vi "Process.vi"(8 "error in":errorcluster, 11 "Inst UI.Framework-Template":refnum<class "Inst UI.Framework-Template.lvclass">) -> (0 "error out":errorcluster, 3 "Inst UI.Framework-Template out":refnum<class "Inst UI.Framework-Template.lvclass">)   [LabVIEW 2019, in "Inst UI.Framework-Template.lvclass"]
doc: "---------------------------------------------------------------\nJKI State Machine Objects™\nhttp://jki.net/state-machine-objects/\nCopyright (C) 2005-2015, JKI <info@jki.net>\nALL RIGHTS RESERVEDJKI State Machine Objects (SMO) 1.0.0.5\nJKI - JKI\nCopyright (c) 2016, JKI"
uses:
  Inst UI.Framework-Template.lvclass
  C:/Program Files (x86)/National Instruments/LabVIEW 2019/vi.lib/JKI/JKI SMO/SMO/SMO.lvclass
  C:/Program Files (x86)/National Instruments/LabVIEW 2019/user.lib/LevyLab/Instrument Framework/SMOs/Instrument UI/Instrument UI.lvclass
  C:/Program Files (x86)/National Instruments/LabVIEW 2019/vi.lib/JKI/JKI SMO/SMO.UI/SMO.UI.lvclass
  Inst.Framework-Template/Typedefs/Inst.Framework-Template.getAll--Cluster.ctl
  Inst.Framework-Template/Inst.Framework-Template.lvclass
  C:/Program Files (x86)/National Instruments/LabVIEW 2019/user.lib/LevyLab/Instrument Framework/SMOs/Instrument/Instrument.lvclass
  Inst UI.Framework-Template.UI--Cluster.ctl
  Inst.Framework-Template/Typedefs/Inst.Framework-Template.Configuration--Cluster.ctl
  <userlib>/LevyLab/Instrument Framework/SMOs/Configuration/Configuration.lvclass
  <userlib>/LevyLab/Instrument Framework/SMOs/RemoteControl/Typedefs/Message--Cluster.ctl
  <userlib>/LevyLab/Instrument Framework/SMOs/Instrument UI/Instrument UI.lvclass/Instrument UI.ctl
  Inst.Framework-Template/Inst.Framework-Template.lvclass/Inst.Framework-Template.ctl
  <vilib>/JKI/JKI SMO/SMO/SMO.lvclass/SMO.ctl
  <userlib>/LevyLab/Instrument Framework/SMOs/Configuration/Configuration.lvclass/Configuration.ctl
  <userlib>/LevyLab/Instrument Framework/SMOs/Instrument/Instrument.lvclass/Instrument.ctl
  <userlib>/LevyLab/Instrument Framework/SMOs/Instrument/Typedefs/Client Type--Enum.ctl
  09e9697b-516c-49fb-b2dc-692589121b6f.vi
  <vilib>/JKI/JKI SMO/SMO/Private/ReftoDVR--SMO.vi
  09e9697b-516c-49fb-b2dc-692589121b6f.vi/e95de145-570b-4452-909a-60166876b235.vi
  09e9697b-516c-49fb-b2dc-692589121b6f.vi/e95de145-570b-4452-909a-60166876b235.vi/36141e6f-c45c-4e10-a95a-9d5fe44f6ec9.vi
  <userlib>/LevyLab/Instrument Framework/SMOs/Instrument/API/Send and Receive.vi
  09e9697b-516c-49fb-b2dc-692589121b6f.vi/e95de145-570b-4452-909a-60166876b235.vi/d03f3c8e-ad6b-4901-9eeb-1b6090619d7a.vi
  <userlib>/LevyLab/Instrument Framework/SMOs/Instrument/Private/Get Client Type.vi
  09e9697b-516c-49fb-b2dc-692589121b6f.vi/e95de145-570b-4452-909a-60166876b235.vi/36141e6f-c45c-4e10-a95a-9d5fe44f6ec9.vi/b5a0ba1c-4e26-4f74-85d6-dad422d985a8.vi
  09e9697b-516c-49fb-b2dc-692589121b6f.vi/e95de145-570b-4452-909a-60166876b235.vi/36141e6f-c45c-4e10-a95a-9d5fe44f6ec9.vi/dc30b0cd-235f-497b-abf4-218ba0e13130.vi
  09e9697b-516c-49fb-b2dc-692589121b6f.vi/e95de145-570b-4452-909a-60166876b235.vi/d03f3c8e-ad6b-4901-9eeb-1b6090619d7a.vi/65f50c0c-55d1-4f0e-9c2f-0837c701ede4.vi
  09e9697b-516c-49fb-b2dc-692589121b6f.vi/e95de145-570b-4452-909a-60166876b235.vi/d03f3c8e-ad6b-4901-9eeb-1b6090619d7a.vi/7c5fe90f-b0b4-4563-867a-64d0d40b5a7e.vi
  09e9697b-516c-49fb-b2dc-692589121b6f.vi/e95de145-570b-4452-909a-60166876b235.vi/d03f3c8e-ad6b-4901-9eeb-1b6090619d7a.vi/65f50c0c-55d1-4f0e-9c2f-0837c701ede4.vi/de2124e9-4285-4bb7-980b-98fcc6874339.vi
  09e9697b-516c-49fb-b2dc-692589121b6f.vi/e95de145-570b-4452-909a-60166876b235.vi/d03f3c8e-ad6b-4901-9eeb-1b6090619d7a.vi/65f50c0c-55d1-4f0e-9c2f-0837c701ede4.vi/669ede32-d20a-4276-b19a-110da03bbeaf.vi
  <userlib>/LevyLab/Instrument Framework/SMOs/Instrument/Private/Get RC Connection Status.vi
  <userlib>/LevyLab/Instrument Framework/SMOs/Instrument/API/Enum to String.vi
  <userlib>/LevyLab/Instrument Framework/SMOs/RemoteControl/API/Send and Receive.vi
  <vilib>/Utility/Data Type/Get Type Information.vi
  <vilib>/JDP Science/JSONtext/JSON text to Variant.vi
  <vilib>/JDP Science/JSONtext/Variant to JSON Text.vi
  <vilib>/National Instruments/GUID Generator/Guid Generator.vi
  <userlib>/LevyLab/Instrument Framework/SMOs/Instrument/Private/Instrument.MessageFromProcess.EventStructure.vi
  <userlib>/LevyLab/Instrument Framework/SMOs/Instrument/Instrument.lvclass
  <vilib>/JDP Science/JSONtext/LVClass Serializer/JSONtext LVClass Serializer.lvclass
  <userlib>/LevyLab/Instrument Framework/SMOs/Instrument UI/Instrument UI.lvclass
  <vilib>/JKI/JKI SMO/SMO/SMO.lvclass
  <vilib>/JKI/JKI SMO/SMO.UI/SMO.UI.lvclass
  <userlib>/LevyLab/Instrument Framework/SMOs/RemoteControl/RemoteControl.lvclass
panel:
  in  "Parameter 2":string
  out "Numeric":u32
  in  "Set Parameter":bool
  in  "Parameter":dbl
  in  "STOP":bool
  out "SMO string":string
  out "SMO Boolean":bool
  out "Logger SMO":dbl
  out "Levy 1":dbl
  # "#todo\nmake UI here. maybe include a nice picture of the hardware?"
  # "#todo\nadd buttons to do stuff (e.g., change a setting)\nButtons should trigger an event"
  # "#todo\nresize this box if you want your UI to be different size"
  # "SMO UI Template"
  # "For instructions on how to use the JKI State Machine Objects, examples and video tutorials, visit:\nhttp://jki.net/state-machine-objects/\n\nJKI State Machine Objects™\nhttp://jki.net/state-machine-objects/\nCopyright (C) 2005-2015, JKI <info@jki.net>\nALL RIGHTS RESERVED"
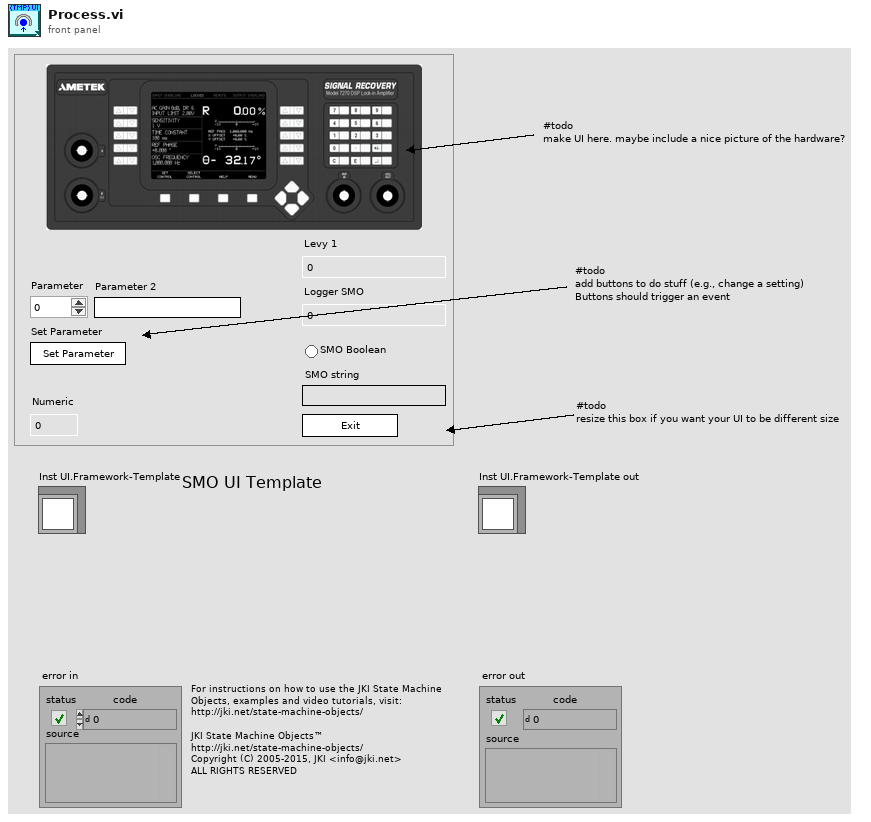
[diagram p1: front panel]
types:
  T1 = enum32{"invalid app kind", "Development System", "Run Time System", "Student Edition", "Embedded LabVIEW", "Evaluation", "Custom"}
  T2 = enum32{"Invalid", "Standard", "Closed", "Hidden", "Minimized", "Maximized"}
  T3 = typedef "Instrument.lvclass/Client Type--Enum.ctl" = enum16{"Remote", "Local"}
  T4 = typedef "Inst.Framework-Template.lvclass/Inst.Framework-Template.Configuration--Cluster.ctl" = cluster{"Example Setting 1":dbl, "Example Setting 2":dbl, "Example Setting 3":string}
  T5 = typedef "Inst.Framework-Template.lvclass/Inst.Framework-Template.getAll--Cluster.ctl" = cluster{"Levy 1":dbl, "Logger SMO":dbl, "SMO Boolean":bool, "SMO String":string}
  T6 = typedef "Inst UI.Framework-Template.lvclass/Inst UI.Framework-Template.UI--Cluster.ctl" = cluster{"Parameter":dbl, "Parameter 2":string}
  T7 = typedef "RemoteControl.lvclass/Message--Cluster.ctl" = cluster{"Command":string, "Data":variant, "ID":string}
  T8 = cluster{"Core":cluster{"Current VI Reference":refnum<vi>, "Close Panel on Exit?":bool, "Last Error":cluster{"error":errorcluster, "previous state":string, "remaining states":string}, "Shutdown?":bool}, "Instrument UI":refnum<class "Inst UI.Framework-Template.lvclass">, "Instrument":refnum<class "Inst.Framework-Template.lvclass">, "Configuration":refnum<class "Configuration.lvclass">, "Config Cluster":T4, "getAll":T5, "UI Cluster":T6, "Message":T7}
  T9 = cluster{"Current VI Reference":refnum<vi>, "Close Panel on Exit?":bool, "Last Error":cluster{"error":errorcluster, "previous state":string, "remaining states":string}, "Shutdown?":bool}
  T10 = typedef "SMO.lvclass/Protected Events.ctl" = cluster{"StopProcesses":refnum<user-event>, "AbortProcesses":refnum<user-event>, "Config Changed":refnum<user-event>, "Dependency":refnum<user-event>}
  T11 = typedef "Instrument.lvclass/PublicEvents--Cluster.ctl" = cluster{"MessageFromProcess":refnum<user-event>}
  T12 = typedef "Inst.Framework-Template.lvclass/PublicEvents--Cluster.ctl" = cluster{"MessageFromProcess":refnum<user-event>}
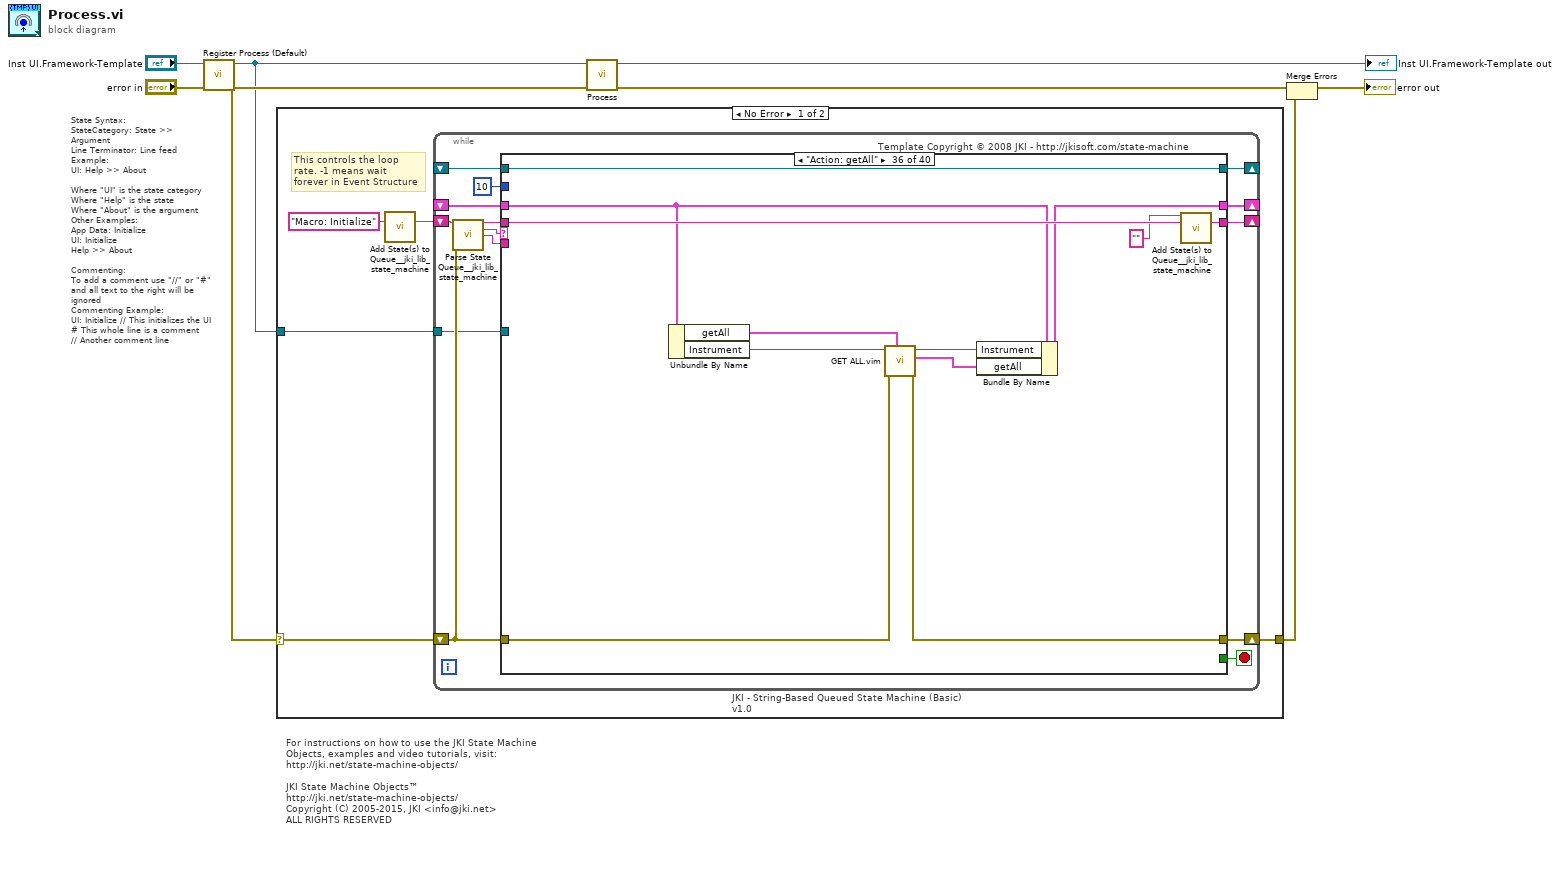
[diagram p0: block diagram]
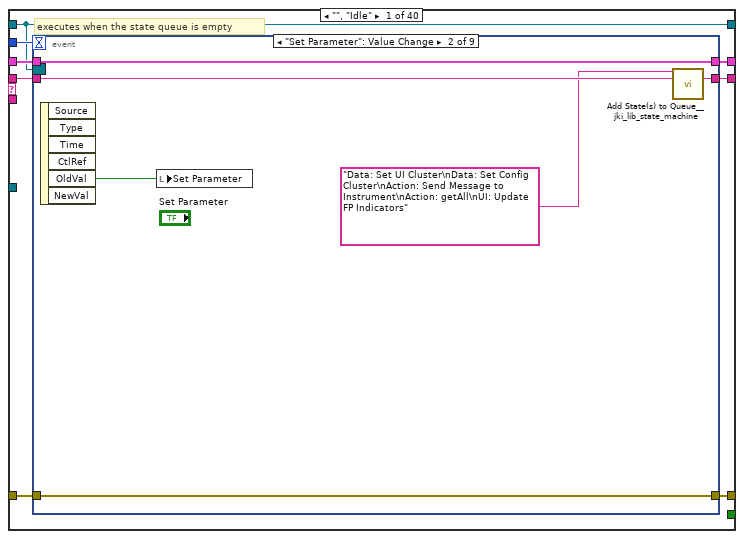
[diagram p2: hidden frame]
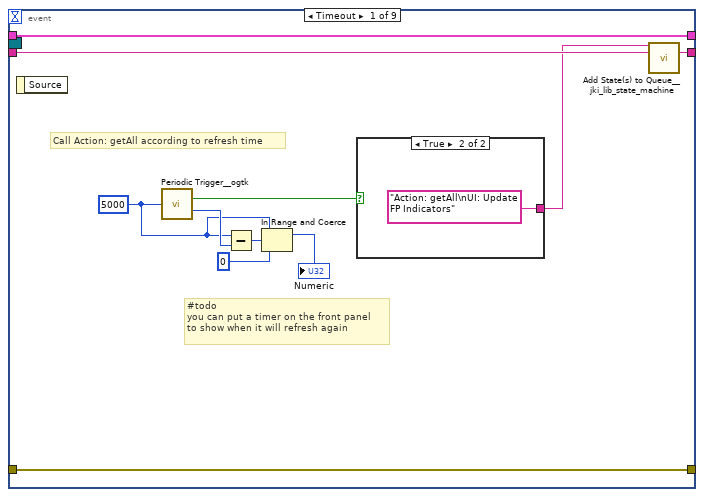
[diagram p3: hidden frame]
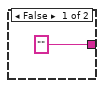
[diagram p4: hidden frame]
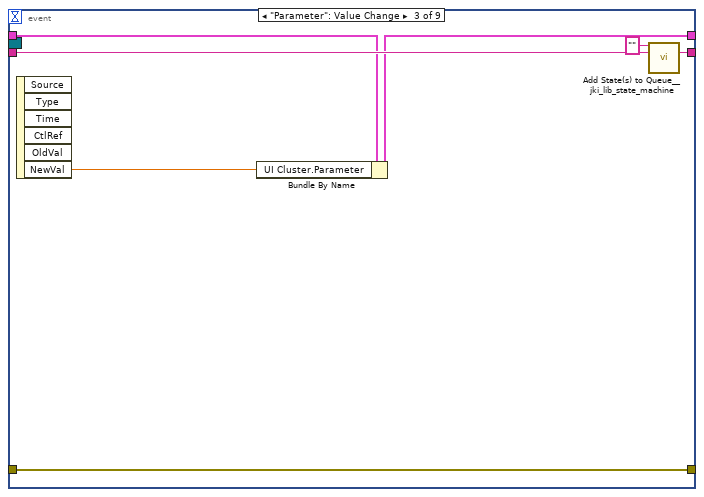
[diagram p5: hidden frame]
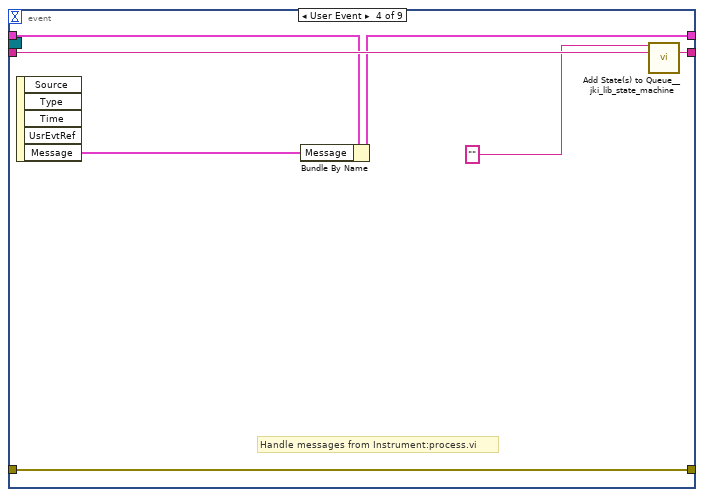
[diagram p6: hidden frame]
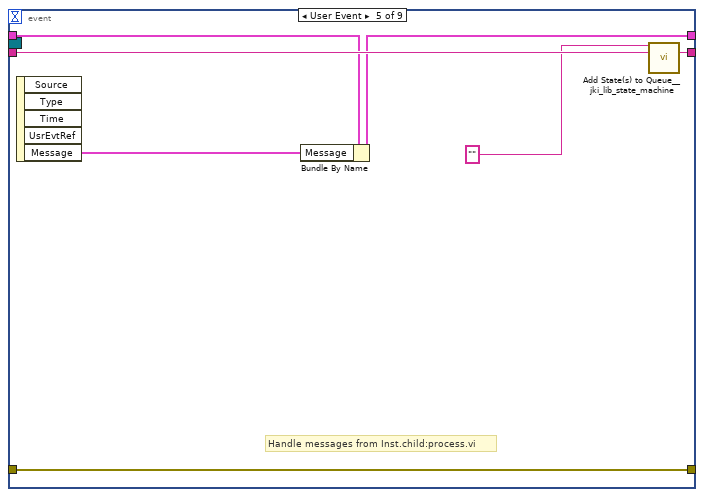
[diagram p7: hidden frame]
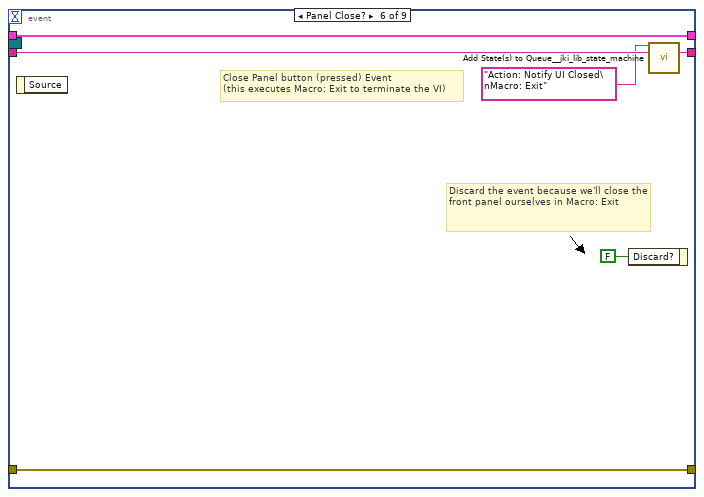
[diagram p8: hidden frame]
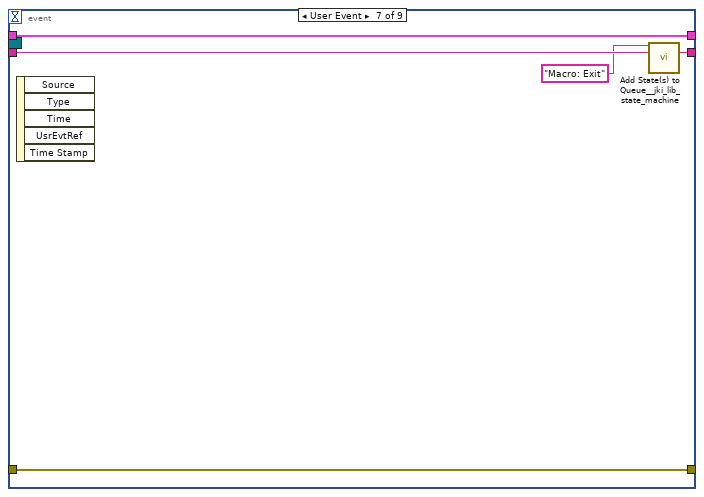
[diagram p9: hidden frame]
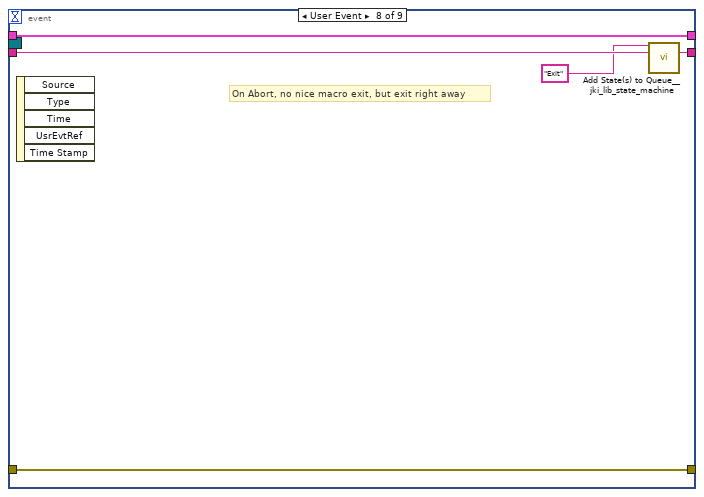
[diagram p10: hidden frame]
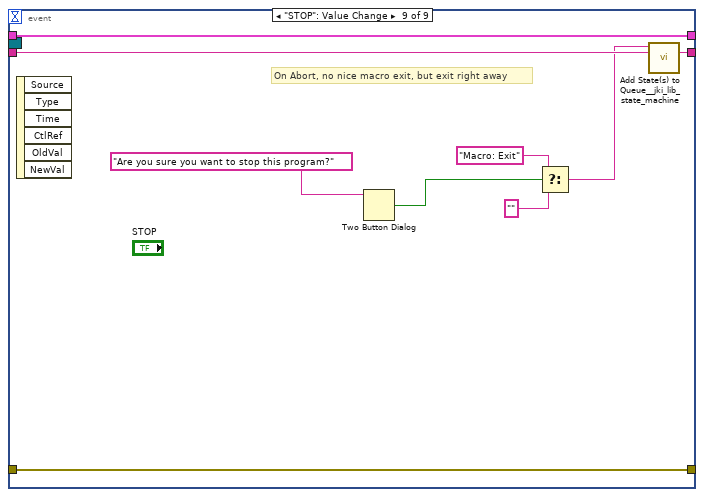
[diagram p11: hidden frame]
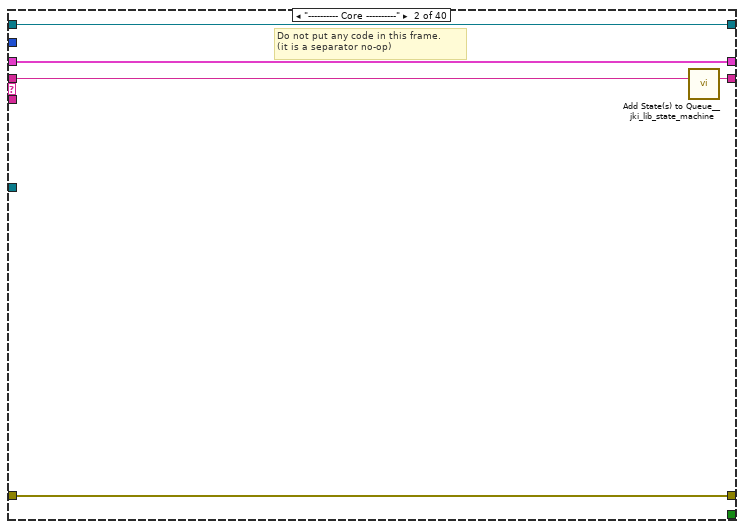
[diagram p12: hidden frame]
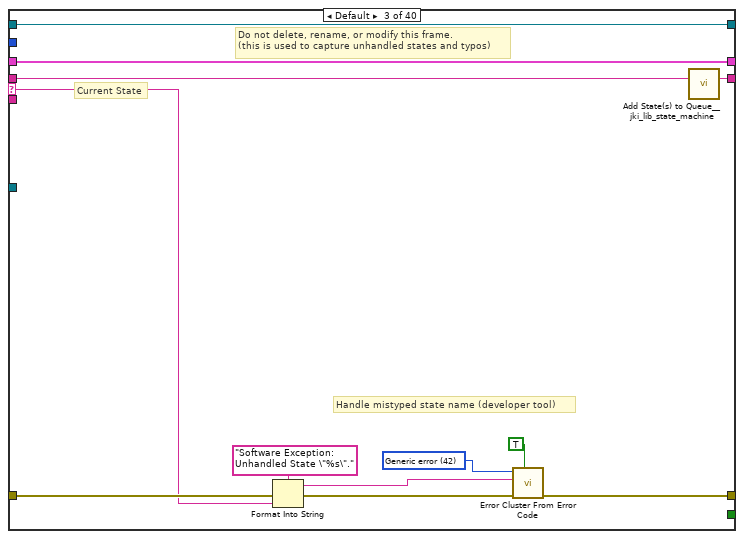
[diagram p13: hidden frame]
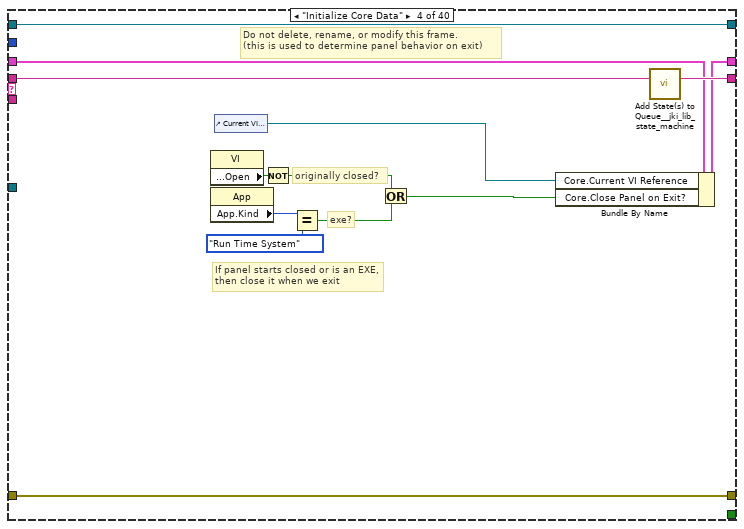
[diagram p14: hidden frame]
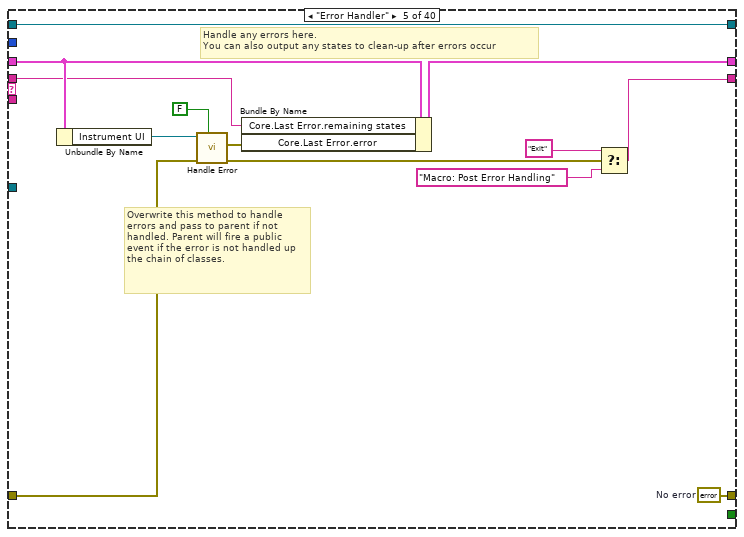
[diagram p15: hidden frame]
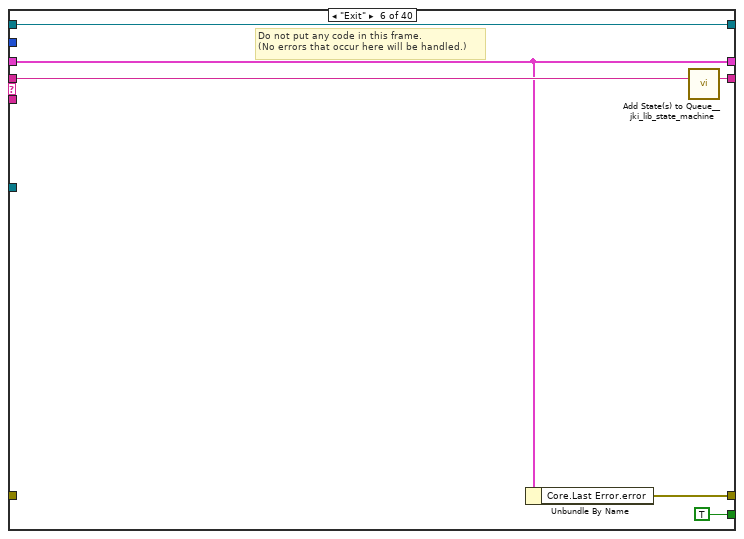
[diagram p16: hidden frame]
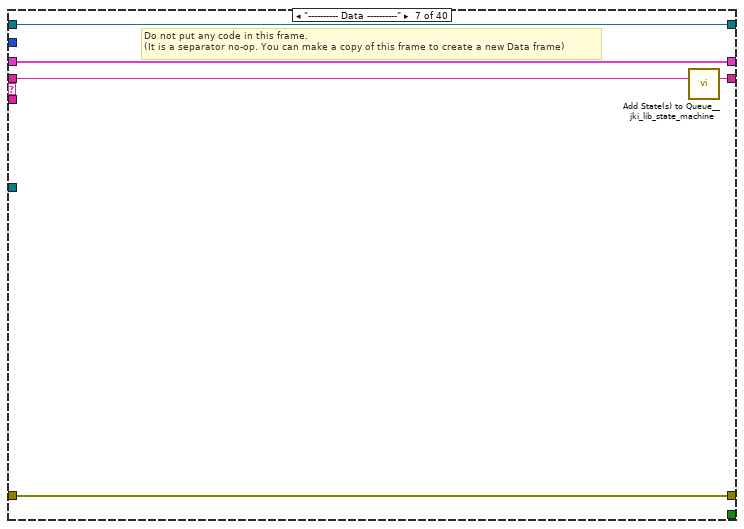
[diagram p17: hidden frame]
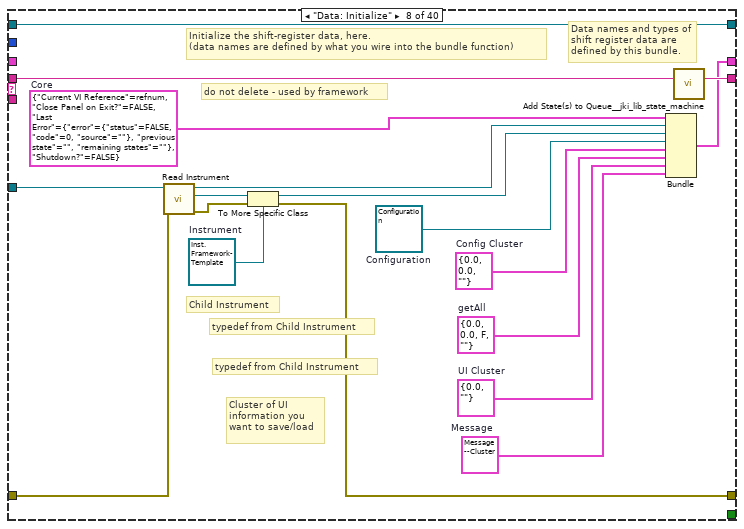
[diagram p18: hidden frame]
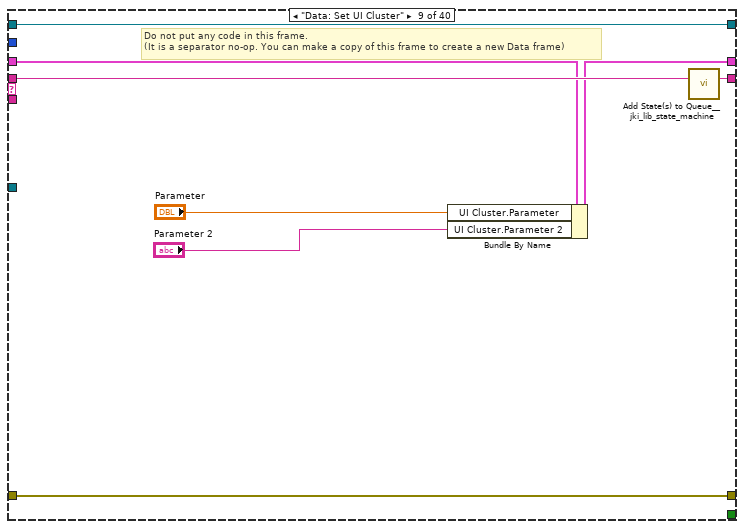
[diagram p19: hidden frame]
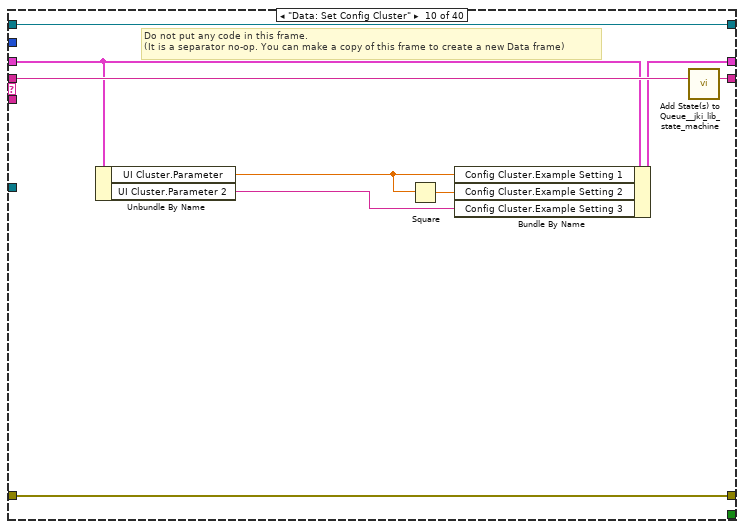
[diagram p20: hidden frame]
diagram:
  # "State Syntax:\nStateCategory: State >> Argument\nLine Terminator: Line feed\nExample:\nUI: Help >> About\n\nWhere \"UI\" is the state category\nWhere \"Help\" is the state\nWhere \"About\" is the argument\nOther Examples:\nApp Data: Initialize\nUI: Initialize\nHelp >> About\n\nCommenting:\nTo add a comment use \"//\" or \"#\" and all text to the right will be ignored\nCommenting Example:\nUI: Initialize // This initializes the UI\n# This whole line is a comment\n// Another comment line"
  # "For instructions on how to use the JKI State Machine Objects, examples and video tutorials, visit:\nhttp://jki.net/state-machine-objects/\n\nJKI State Machine Objects™\nhttp://jki.net/state-machine-objects/\nCopyright (C) 2005-2015, JKI <info@jki.net>\nALL RIGHTS RESERVED"
  n1 = call <vilib>:"Register Process (Default).vi"("error in (no error)"="error in", "SMO"="Inst UI.Framework-Template") -> ("error out"=w5:errorcluster, "SelfRef"=w4:refnum<class "Inst UI.Framework-Template.lvclass">)  [unwired: 8 in]
  n2 = case shown="No Error" w5 {
    selector: w5 -> [w10 w492]
    tunnel: w4 -> [w11 _]
    tunnel: [w9 w492] -> w1
    frame No Error {
      # "This controls the loop rate. -1 means wait forever in Event Structure"
      n3 = call <vilib>:"Add State(s) to Queue__jki_lib_state_machine.vi"("State(s) in (\"\")"="Macro: Initialize") -> ("States Out"=w13:string)  [unwired: 14 in]
      n4 = while "JKI - String-Based Queued State Machine (Basic) v1.0" {
        shift-right: [w20] -> _
        shift-left: _ -> [w19]
        shift-right: [w23] -> w9
        shift-left: w10 -> [w17]
        shift-right: [w22] -> _
        shift-left: w13 -> [w24]
        tunnel: w11 -> [w16]
        shift-right: [w15] -> _
        shift-left: _ -> [w14]
        stop <- w21 stop-if-true
        # "Template Copyright © 2008 JKI - http://jkisoft.com/state-machine"
        n5 = call <vilib>:"Parse State Queue__jki_lib_state_machine.vi"("State Queue"=w24, "Error In (no error)"=w17) -> ("Remaining States"=w26:string, "Current State"=w27:string, "Arguments"=w25:string)  [unwired: 11 in]
        n6 = case shown="\"Action: getAll\"" w27 {
          selector: w27 -> [_ _ w107 _ _ _ _ _ _ _ _ _ _ _ _ _ _ _ _ _ _ _ _ _ _ _ _ _ _ _ _ _ _ _ _ _ _ _ _ _]
          tunnel: w26 -> [w35 w105 w111 w130 w134 w149 w154 w172 w180 w189 w196 w201 w208 w215 w225 w232 w248 w280 w289 w301 w311 w317 w332 w337 w348 w355 w360 w376 w382 w387 w402 w410 w422 w429 w436 w448 w461 w471 w481 w491]
          tunnel: w25 -> [_ _ _ _ _ _ _ _ _ _ _ _ _ _ _ w226 w242 _ _ _ _ _ _ _ _ _ _ _ _ _ _ _ _ _ _ _ _ _ _ _]
          tunnel: w19 -> [w33 w102 w109 w121 w137 w145 w151 _ w176 w185 w190 w198 w206 w211 w216 w230 w244 w277 w285 w291 w308 w314 w319 w334 w345 w350 w357 w374 w380 w384 w395 w407 w413 w424 w430 w440 w455 w463 w476 w486]
          tunnel: [w32 w103 w113 w127 w139 w144 w152 w159 w178 w187 w192 w199 w203 w213 w217 w227 w245 w278 w287 w299 w309 w315 w330 w335 w339 w351 w358 w371 w377 w385 w388 w405 w414 w426 w431 w445 w458 w468 w472 w482] -> w23
          tunnel: w17 -> [w31 w103 w112 w127 w133 _ w152 w156 w178 w187 w193 w199 w204 w213 w217 w228 w246 w278 w287 w299 w309 w315 w330 w335 w340 w352 w358 w361 w378 w385 w397 w403 w415 w426 w432 w441 w450 w464 w473 w483]
          tunnel: [w34 w104 w110 w129 w131 w148 w153 w171 w179 w188 w195 w200 w207 w214 w224 w231 w247 w279 w288 w300 w310 w316 w331 w336 w347 w354 w359 w375 w381 w386 w401 w409 w421 w428 w435 w447 w460 w470 w480 w490] -> w22
          tunnel: [_ _ _ _ _ TRUE _ _ _ _ _ _ _ _ _ _ _ _ _ _ _ _ _ _ _ _ _ _ _ _ _ _ _ _ _ _ _ _ _ _] -> w21
          tunnel: [w30 w102 w109 w128 w136 w145 w151 w170 w175 w184 w190 w198 w206 w211 w216 w230 w244 w277 w285 w292 w308 w314 w319 w334 w345 w350 w357 w374 w380 w384 w399 w407 w411 w423 w430 w442 w456 w465 w477 w487] -> w20
          tunnel: 10 ("Timeout") -> [w29 _ _ _ _ _ _ _ _ _ _ _ _ _ _ _ _ _ _ _ _ _ _ _ _ _ _ _ _ _ _ _ _ _ _ _ _ _ _ _]
          tunnel: w16 -> [_ _ _ _ _ _ _ w157 _ _ _ _ _ _ _ _ _ _ _ _ _ _ _ _ _ _ _ _ _ _ _ _ _ _ _ _ _ _ _ _]
          tunnel: [w28 w101 w106 w118 w143 w146 w150 w169 w177 w186 w191 w197 w205 w212 w223 w229 w241 w276 w286 w298 w307 w313 w324 w333 w346 w353 w356 w373 w379 w383 w400 w408 w420 w427 w434 w446 w459 w469 w479 w489] -> w15
          tunnel: w14 -> [w28 w101 w106 w118 w143 w146 w150 w169 w177 w186 w191 w197 w205 w212 w223 w229 w241 w276 w286 w298 w307 w313 w324 w333 w346 w353 w356 _ w379 w383 w400 w408 w420 w427 w434 w446 w459 w469 w479 w489]
          frame "", "Idle" {
            # "executes when the state queue is empty"
            n7 = event shown="[1] \"Set Parameter\": Value Change" {
              selector: w28 -> [_ _ _ _ _ _ _ _ _]
              dyn-events: _ -> [_ _ _ _ _ _ _ _ _]
              timeout: w29 -> [_ _ _ _ _ _ _ _ _]
              tunnel: w35 -> [w46 w54 w61 w68 w75 w81 w86 w91 w100]
              tunnel: [w45 w53 w60 w67 w74 w80 w85 w90 w99] -> w34
              tunnel: w33 -> [w43 w51 w57 w65 w72 w77 w83 w88 w97]
              tunnel: [w44 w52 w59 w66 w73 w76 w84 w89 w98] -> w32
              tunnel: w31 -> [w44 w52 w59 w66 w73 w76 w84 w89 w98]
              tunnel: [w43 w51 w56 w64 w71 w77 w83 w88 w97] -> w30
              event Timeout {
                w37 = u32 5000 ("time (ms)")
                # "#todo\nyou can put a timer on the front panel\nto show when it will refresh again"
                # "Call Action: getAll according to refresh time"
                n8 = event-data() -> ()  [unwired: 1 in, 1 out]
                n9 = call <userlib>:"Periodic Trigger__ogtk.vi"("time (ms)"=w37) -> ("Triggered"=w41:bool, "timer value"=w40:u32)  [unwired: 12 in, 1 out]
                n10 = Subtract(x=w37, y=w40) -> (x-y=w39:u32)
                n11 = In Range and Coerce(upper limit=w37, x=w39, lower limit=u32 0) -> (coerced(x)=→"Numeric":u32)  [unwired: 1 out]
                n12 = case shown="True" w41 {
                  tunnel: ["" ("State(s) in Front (\"\")") "Action: getAll\nUI: Update FP Indicators" ("State(s) in Front (\"\")")] -> w42
                  frame False {
                  }
                  frame True {
                  }
                }
                n13 = call <vilib>:"Add State(s) to Queue__jki_lib_state_machine.vi"("State(s) in Front (\"\")"=w42, "State(s) in (\"\")"=w46) -> ("States Out"=w45:string)  [unwired: 13 in]
              }
              event "Set Parameter": Value Change {
                n14 = event-data() -> ("OldVal"=w50:bool)  [unwired: 1 in, 5 out]
                n15 = local write "Set Parameter"(w50) -> ()
                n16 = call <vilib>:"Add State(s) to Queue__jki_lib_state_machine.vi"("State(s) in Front (\"\")"="Data: Set UI Cluster\nData: Set Config Cluster\nAction: Send Message to Instrument\nAction: getAll\nUI: Update FP Indicators" ("State(s) in Front (\"\")"), "State(s) in (\"\")"=w54) -> ("States Out"=w53:string)  [unwired: 13 in]
              }
              event "Parameter": Value Change {
                n17 = event-data() -> ("NewVal"=w58:dbl)  [unwired: 1 in, 5 out]
                n18 = Bundle By Name(cluster=w57, "UI Cluster.Parameter"=w58) -> (w56:T8)
                n19 = call <vilib>:"Add State(s) to Queue__jki_lib_state_machine.vi"("State(s) in Front (\"\")"="" ("State(s) in Front (\"\")"), "State(s) in (\"\")"=w61) -> ("States Out"=w60:string)  [unwired: 13 in]
              }
              event User Event {
                # "Handle messages from Instrument:process.vi"
                n20 = event-data() -> ("Message"=w62:T7)  [unwired: 1 in, 4 out]
                n21 = Bundle By Name(cluster=w65, "Message"=w62) -> (w64:T8)
                n22 = call <vilib>:"Add State(s) to Queue__jki_lib_state_machine.vi"("State(s) in Front (\"\")"="" ("State(s) in Front (\"\")"), "State(s) in (\"\")"=w68) -> ("States Out"=w67:string)  [unwired: 13 in]
              }
              event User Event {
                # "Handle messages from Inst.child:process.vi"
                n23 = event-data() -> ("Message"=w69:T7)  [unwired: 1 in, 4 out]
                n24 = Bundle By Name(cluster=w72, "Message"=w69) -> (w71:T8)
                n25 = call <vilib>:"Add State(s) to Queue__jki_lib_state_machine.vi"("State(s) in Front (\"\")"="" ("State(s) in Front (\"\")"), "State(s) in (\"\")"=w75) -> ("States Out"=w74:string)  [unwired: 13 in]
              }
              event Panel Close? {
                # "Discard the event because we'll close the front panel ourselves in Macro: Exit"
                # "Close Panel button (pressed) Event\n(this executes Macro: Exit to terminate the VI)"
                n26 = event-data() -> ()  [unwired: 1 in, 1 out]
                n27 = event-data("Discard?"=FALSE) -> ()  [unwired: 1 in, 1 out]
                n28 = call <vilib>:"Add State(s) to Queue__jki_lib_state_machine.vi"("State(s) in Front (\"\")"="Action: Notify UI Closed\nMacro: Exit", "State(s) in (\"\")"=w81) -> ("States Out"=w80:string)  [unwired: 13 in]
              }
              event User Event {
                n29 = event-data() -> ()  [unwired: 1 in, 5 out]
                n30 = call <vilib>:"Add State(s) to Queue__jki_lib_state_machine.vi"("State(s) in Front (\"\")"="Macro: Exit", "State(s) in (\"\")"=w86) -> ("States Out"=w85:string)  [unwired: 13 in]
              }
              event User Event {
                # "On Abort, no nice macro exit, but exit right away"
                n31 = event-data() -> ()  [unwired: 1 in, 5 out]
                n32 = call <vilib>:"Add State(s) to Queue__jki_lib_state_machine.vi"("State(s) in Front (\"\")"="Exit", "State(s) in (\"\")"=w91) -> ("States Out"=w90:string)  [unwired: 13 in]
              }
              event "STOP": Value Change {
                # "On Abort, no nice macro exit, but exit right away"
                n33 = event-data() -> ()  [unwired: 1 in, 6 out]
                n34 = Two Button Dialog(message="Are you sure you want to stop this program?") -> (T button?=w96:bool)  [unwired: 2 in]
                n35 = Select(t="Macro: Exit", s=w96, f="") -> (s? t:f=w92:string)
                n36 = call <vilib>:"Add State(s) to Queue__jki_lib_state_machine.vi"("State(s) in Front (\"\")"=w92, "State(s) in (\"\")"=w100) -> ("States Out"=w99:string)  [unwired: 13 in]
              }
            }
          }
          frame "---------- Core ----------" {
            # "Do not put any code in this frame.\n(it is a separator no-op)"
            n37 = call <vilib>:"Add State(s) to Queue__jki_lib_state_machine.vi"("State(s) in (\"\")"=w105) -> ("States Out"=w104:string)  [unwired: 14 in]
          }
          frame Default {
            w116 = 42 items=["No error", "Argument error", "Memory is full", "Out of zone", "End of file", "File already open", "Generic file I/O error", "File not found", "File permission error", "Disk is full", "Duplicate path", "Too many files open", "System feature not enabled", "Resource file not found", "Cannot add resource", "Resource not found", "Image not found", "Image memory error", "Pen does not exist", "Config type invalid", "Config token not found", "Config parse error", "Config memory error", "Bad external code format", "Bad external code offset", "External code not present", "Null window", "Destroy window error", "Null menu", "Print aborted", "Bad print record", "Print driver error", "Windows error during printing", "Memory error during printing", "Print dialog error", "Generic print error", "Invalid device refnum", "Device not found", "Device parameter error", "Device unit error", "Cannot open device", "Device call aborted", "Generic error", "Cancelled by user", "Object ID too low", "Object ID too high", "Object not in heap", "Unknown heap", "Unknown object (invalid DefProc)", "Unknown object (DefProc not in table)", "Message out of range", "Invalid (null) method", "Unknown message", "Manager call not supported", "Bad address", "Network operation in progress", "Network operation timed out", "Connection is busy", "Network attribute not supported", "Network error", "Address in use", "System out of memory", "Connection aborted", "Connection refused", "Not connected", "Already connected", "Connection closed", "Initialization error (interapplication manager)", "Bad occurrence", "Wait on unbound occurrence handler", "Occurrence queue overflow", "Datalog type conflict", "Unused", "Unrecognized type (interapplication manager)", "Memory corrupt", "Failed to make temporary DLL", "Old CIN version", "Drag socket not found", "Failed to load drop-object", "Failed to register OLE object", "Failed to release OLE object", "Format specifier type mismatch", "Unknown format specifier", "Too few format specifiers", "Too many format specifiers", "Scan failed", "Newer CIN version", "Error converting to variant", "Runtime menu error", "Password tampered", "Variant attribute not found", "Incompatible variant data type", "Event data is not available", "Event Store is not present", "Occurrence is not found", "Event Queue is not created", "Event info is not available", "Refnum passed is NULL", "Error retrieving Class GUID", "Error retrieving CoClass GUID", "Error retrieving TypeLib GUID.", "Bad built application magic bytes.", "Specific driver is different from the specific driver associated with the Logical Name.", "There is no session opened to the class driver.", "Max Error", "MAX - Error with config objects", "MAX - Error loading configuration", "MAX - Group not supported"]
            # "Current State"
            # "Do not delete, rename, or modify this frame.\n(this is used to capture unhandled states and typos)"
            # "Handle mistyped state name (developer tool)"
            n38 = Format Into String(format string="Software Exception: Unhandled State \"%s\"." ("message"), error in=w112, w107) -> (resulting string=w115:string, error out=w114:errorcluster)  [unwired: 1 in]
            n39 = call <vilib>:"Error Cluster From Error Code.vi"("show call chain? (False)"=TRUE, "error in (no error)"=w114, "error message (\"\")"=w115, "error code (0)"=w116) -> ("error out"=w113:errorcluster)  [unwired: 5 in]
            n40 = call <vilib>:"Add State(s) to Queue__jki_lib_state_machine.vi"("State(s) in (\"\")"=w111) -> ("States Out"=w110:string)  [unwired: 14 in]
          }
          frame "Initialize Core Data" {
            # "Do not delete, rename, or modify this frame.\n(this is used to determine panel behavior on exit)"
            # "originally closed?"
            # "exe?"
            # "If panel starts closed or is an EXE, then close it when we exit"
            n41 = property class="VI"() -> ("Front Panel.Open"=w126:bool)  [unwired: 2 in, 2 out]
            n42 = property class="App"() -> ("App.Kind"=w125:T1)  [unwired: 2 in, 2 out]
            n43 = control-ref of="Current VI Reference"() -> (w119:refnum<vi>)
            n44 = Not(x=w126) -> (.not. x?=w123:bool)
            n45 = Equal?(x=w125, y=T1."Run Time System" ("Application:Kind")) -> (x = y?=w122:bool)
            n46 = Or(x=w123, y=w122) -> (x .or. y?=w120:bool)
            n47 = Bundle By Name(cluster=w121, "Core.Current VI Reference"=w119, "Core.Close Panel on Exit?"=w120) -> (w128:T8)
            n48 = call <vilib>:"Add State(s) to Queue__jki_lib_state_machine.vi"("State(s) in (\"\")"=w130) -> ("States Out"=w129:string)  [unwired: 14 in]
          }
          frame "Error Handler" {
            w139 = errorcluster {"status"=FALSE, "code"=0, "source"=""}  # No error
            # "Overwrite this method to handle errors and pass to parent if not handled. Parent will fire a public event if the error is not handled up the chain of classes."
            # "Handle any errors here.\nYou can also output any states to clean-up after errors occur"
            n49 = Unbundle By Name(w137) -> ("Instrument UI"=w142:refnum<class "Inst UI.Framework-Template.lvclass">)
            n50 = call-dynamic "Handle Error.vi"("Stop on Unhandled Error (T)"=FALSE, "error in"=w133, "SMO"=w142) -> ("handling error"=w140:errorcluster, "Unhandled error"=w138:errorcluster)  [unwired: 6 in, 1 out]
            n51 = Bundle By Name(cluster=w137, "Core.Last Error.remaining states"=w134, "Core.Last Error.error"=w138) -> (w136:T8)
            n52 = Select(t="Exit", s=w140, f="Macro: Post Error Handling") -> (s? t:f=w131:string)
          }
          frame "Exit" {
            # "Do not put any code in this frame.\n(No errors that occur here will be handled.)"
            n53 = Unbundle By Name(w145) -> ("Core.Last Error.error"=w144:errorcluster)
            n54 = call <vilib>:"Add State(s) to Queue__jki_lib_state_machine.vi"("State(s) in (\"\")"=w149) -> ("States Out"=w148:string)  [unwired: 14 in]
          }
          frame "---------- Data ----------" {
            # "Do not put any code in this frame.\n(It is a separator no-op. You can make a copy of this frame to create a new Data frame)"
            n55 = call <vilib>:"Add State(s) to Queue__jki_lib_state_machine.vi"("State(s) in (\"\")"=w154) -> ("States Out"=w153:string)  [unwired: 14 in]
          }
          frame "Data: Initialize" {
            w155 = T7 {"Command"="", "Data"=variant, "ID"=""}  # Message
            w158 = refnum<class "Configuration.lvclass"> refnum  # Configuration
            w161 = T4 {"Example Setting 1"=0.0, "Example Setting 2"=0.0, "Example Setting 3"=""}  # Config Cluster
            w163 = T6 {"Parameter"=0.0, "Parameter 2"=""}  # UI Cluster
            w165 = refnum<class "Inst.Framework-Template.lvclass"> refnum  # Instrument
            w167 = T5 {"Levy 1"=0.0, "Logger SMO"=0.0, "SMO Boolean"=FALSE, "SMO String"=""}  # getAll
            w168 = T9 {"Current VI Reference"=refnum, "Close Panel on Exit?"=FALSE, "Last Error"={"error"={"status"=FALSE, "code"=0, "source"=""}, "previous state"="", "remaining states"=""}, "Shutdown?"=FALSE}  # Core
            # "typedef from Child Instrument"
            # "Cluster of UI\ninformation you\nwant to save/load"
            # "Child Instrument"
            # "typedef from Child Instrument"
            # "do not delete - used by framework"
            # "Data names and types of shift register data are defined by this bundle."
            # "Initialize the shift-register data, here.\n(data names are defined by what you wire into the bundle function)"
            n56 = call <userlib>:"Read Instrument.vi"("error in (no error)"=w156, "Instrument UI in"=w157) -> ("error out"=w162:errorcluster, "Instrument"=w164:refnum<class "Instrument.lvclass">, "Instrument UI"=w166:refnum<class "Inst UI.Framework-Template.lvclass">)  [unwired: 7 in]
            n57 = To More Specific Class(target class=w165, reference=w164, error in=w162) -> (specific class reference=w160:refnum<class "Inst.Framework-Template.lvclass">, error out=w159:errorcluster)
            n58 = Bundle("Core"=w168, "Instrument UI"=w166, "Instrument"=w160, "Configuration"=w158, "Config Cluster"=w161, "getAll"=w167, "UI Cluster"=w163, "Message"=w155) -> (w170:T8)  [unwired: 1 in]
            n59 = call <vilib>:"Add State(s) to Queue__jki_lib_state_machine.vi"("State(s) in (\"\")"=w172) -> ("States Out"=w171:string)  [unwired: 14 in]
          }
          frame "Data: Set UI Cluster" {
            # "Do not put any code in this frame.\n(It is a separator no-op. You can make a copy of this frame to create a new Data frame)"
            n60 = Bundle By Name(cluster=w176, "UI Cluster.Parameter"="Parameter", "UI Cluster.Parameter 2"="Parameter 2") -> (w175:T8)
            n61 = call <vilib>:"Add State(s) to Queue__jki_lib_state_machine.vi"("State(s) in (\"\")"=w180) -> ("States Out"=w179:string)  [unwired: 14 in]
          }
          frame "Data: Set Config Cluster" {
            # "Do not put any code in this frame.\n(It is a separator no-op. You can make a copy of this frame to create a new Data frame)"
            n62 = Unbundle By Name(w185) -> ("UI Cluster.Parameter"=w182:dbl, "UI Cluster.Parameter 2"=w183:string)
            n63 = Square(x=w182) -> (x^2=w181:dbl)
            n64 = Bundle By Name(cluster=w185, "Config Cluster.Example Setting 1"=w182, "Config Cluster.Example Setting 2"=w181, "Config Cluster.Example Setting 3"=w183) -> (w184:T8)
            n65 = call <vilib>:"Add State(s) to Queue__jki_lib_state_machine.vi"("State(s) in (\"\")"=w189) -> ("States Out"=w188:string)  [unwired: 14 in]
          }
          frame "Data: Cleanup" {
            # "Cleanup any data and references, here.\n(this is called automatically, by the Macro: Exit)"
            n66 = Unbundle By Name(w190) -> ("Core.Current VI Reference"=w194:refnum<vi>)
            n67 = Close Reference(reference=w194, error in (no error)=w193) -> (error out=w192:errorcluster)
            n68 = call <vilib>:"Add State(s) to Queue__jki_lib_state_machine.vi"("State(s) in (\"\")"=w196) -> ("States Out"=w195:string)  [unwired: 14 in]
          }
          frame "---------- UI ----------" {
            # "Do not put any code in this frame.\n(It is a separator no-op. You can make a copy of this frame to create a new UI frame)"
            n69 = call <vilib>:"Add State(s) to Queue__jki_lib_state_machine.vi"("State(s) in (\"\")"=w201) -> ("States Out"=w200:string)  [unwired: 14 in]
          }
          frame "UI: Initialize" {
            # "size window to decoration box on front panel"
            # "Initialize the User Interface, here.\n(this is called automatically, by the Macro: Init)"
            n70 = invoke on="STOP" class="Bool (strict)" method="Reinit To Default"() -> ()  [unwired: 3 in, 3 out]
            n71 = call <userlib>:"Fit VI window to Largest Dec__ogtk.vi"("error in (no error)"=w204, "border spacing (2 px)"=0) -> ("error out"=w203:errorcluster)  [unwired: 4 in, 1 out]
            n72 = call <vilib>:"Add State(s) to Queue__jki_lib_state_machine.vi"("State(s) in (\"\")"=w208) -> ("States Out"=w207:string)  [unwired: 14 in]
          }
          frame "UI: Update FP Controls" {
            # "Do not put any code in this frame.\n(It is a separator no-op. You can make a copy of this frame to create a new UI frame)"
            n73 = Unbundle By Name(w211) -> ("UI Cluster.Parameter"=w209:dbl, "UI Cluster.Parameter 2"=w210:string)
            n74 = local write "Parameter 2"(w210) -> ()
            n75 = local write "Parameter"(w209) -> ()
            n76 = call <vilib>:"Add State(s) to Queue__jki_lib_state_machine.vi"("State(s) in (\"\")"=w215) -> ("States Out"=w214:string)  [unwired: 14 in]
          }
          frame "UI: Update FP Indicators" {
            # "do this way to have nicer UI or only display what you want"
            n77 = Unbundle By Name(w216) -> ("getAll"=w218:T5)
            n78 = Unbundle By Name(w218) -> ("Levy 1"=→"Levy 1":dbl, "Logger SMO"=→"Logger SMO":dbl, "SMO Boolean"=→"SMO Boolean":bool, "SMO String"=→"SMO string":string)
            n79 = call <vilib>:"Add State(s) to Queue__jki_lib_state_machine.vi"("State(s) in (\"\")"=w225) -> ("States Out"=w224:string)  [unwired: 14 in]
          }
          frame "UI: Cursor Set" {
            # "Argument"
            # "Initialize the User Interface, here.\n(this is called automatically, by the Macro: Init)"
            n80 = disable-structure shown="Default" {
              disable-tunnel: w228 -> [w233 w236]
              disable-tunnel: [w233 w235] -> w227
              disable-tunnel: w226 -> [_ w234]
              frame condition #0 {
              }
              frame condition #1 (active) {
                n81 = case shown="\"Busy\"" w234 {
                  tunnel: w236 -> [w238 w240]
                  tunnel: [w237 w239] -> w235
                  frame "Idle", Default {
                    n82 = call <vilib>:"Unset Busy.vi"("error in (no error)"=w238) -> ("error out"=w237:errorcluster)  [unwired: 10 in]
                  }
                  frame "Busy" {
                    n83 = call <vilib>:"Set Busy.vi"("error in (no error)"=w240) -> ("error out"=w239:errorcluster)  [unwired: 9 in, 1 out]
                  }
                }
              }
            }
            n84 = call <vilib>:"Add State(s) to Queue__jki_lib_state_machine.vi"("State(s) in (\"\")"=w232) -> ("States Out"=w231:string)  [unwired: 14 in]
          }
          frame "UI: Front Panel State" {
            # "Argument"
            # "Set Front Panel Open or Closed\n(Usage: \"UI: Front Panel State >> Open|Close\")"
            n85 = Unbundle By Name(w244) -> ("Core.Current VI Reference"=w243:refnum<vi>)
            n86 = disable-structure shown="Default" {
              disable-tunnel: w246 -> [w252 w275]
              disable-tunnel: [w251 w275] -> w245
              disable-tunnel: w243 -> [w250 _]
              disable-tunnel: w242 -> [w249 _]
              frame condition #0 (active) {
                n87 = case shown="\"Close\"" w249 {
                  tunnel: w252 -> [w256 w269]
                  tunnel: [w258 w270] -> w251
                  tunnel: w250 -> [w257 w267]
                  frame "Open", Default {
                    n88 = property class="VI"(reference=w257, error in=w256) -> (reference out=w254:refnum<vi>, error out=w255:errorcluster, "FP.State"=w253:T2)
                    n89 = case shown="\"Closed\"" w253 {
                      tunnel: [w261 w264] -> w258
                      tunnel: w255 -> [w260 w264]
                      tunnel: w254 -> [w259 _]
                      frame "Closed" {
                        n90 = invoke class="VI" method="FP.Open"(reference=w259, error in=w260, "Activate"=TRUE, "State"=T2."Standard") -> (error out=w261:errorcluster)  [unwired: 1 in, 4 out]
                      }
                      frame Default {
                      }
                    }
                  }
                  frame "Close" {
                    n91 = property class="VI"(reference=w267, error in=w269) -> (reference out=w266:refnum<vi>, error out=w268:errorcluster, "FP.State"=w265:T2)
                    n92 = case shown="Default" w265 {
                      tunnel: [w271 w274] -> w270
                      tunnel: w268 -> [w271 w273]
                      tunnel: w266 -> [_ w272]
                      frame "Invalid", "Closed" {
                      }
                      frame Default {
                        n93 = invoke class="VI" method="FP.Close"(reference=w272, error in=w273) -> (error out=w274:errorcluster)  [unwired: 1 in, 2 out]
                      }
                    }
                  }
                }
              }
              frame condition #1 {
              }
            }
            n94 = call <vilib>:"Add State(s) to Queue__jki_lib_state_machine.vi"("State(s) in (\"\")"=w248) -> ("States Out"=w247:string)  [unwired: 14 in]
          }
          frame "---------- Macro ----------" {
            # "Do not put any code in this frame.\n(It is a separator no-op. You can make a copy of this frame to create a new Macro frame)"
            n95 = call <vilib>:"Add State(s) to Queue__jki_lib_state_machine.vi"("State(s) in (\"\")"=w280) -> ("States Out"=w279:string)  [unwired: 14 in]
          }
          frame "Macro: Initialize" {
            w283 = "UI: Initialize\nMacro: Read UI Config\nAction: Open\n//UI: Front Panel State >> Open"  # UI: Initialize Macro: Read UI Config Action: Open //UI: Front Panel State >> Open
            # "Initialization Macro\n(This is called once, when the VI starts)"
            n96 = call <vilib>:"Add State(s) to Queue__jki_lib_state_machine.vi"("State(s) in Front (\"\")"="Data: Initialize\nInitialize Core Data\nEvents: Register", "State(s) in (\"\")"="Process: Sync", "State(s) at Back (\"\")"=w283) -> ("States Out"=w282:string)  [unwired: 12 in]
            n97 = call <vilib>:"Add State(s) to Queue__jki_lib_state_machine.vi"("State(s) in Front (\"\")"=w282, "State(s) in (\"\")"=w289) -> ("States Out"=w288:string)  [unwired: 13 in]
          }
          frame "Macro: Post Error Handling" {
            # "Clear Last Error?"
            n98 = Unbundle By Name(w291) -> ("Core.Last Error.remaining states"=w293:string, "Core.Shutdown?"=w294:bool)
            n99 = Unbundle By Name(w291) -> ("Core.Last Error.error"=w297:errorcluster)
            n100 = case shown="False" FALSE {
              tunnel: w297 -> [w305 _]
              tunnel: [w305 _] -> w296
              frame False {
              }
              frame True {
              }
            }
            n101 = case shown="True" w294 {
              tunnel: w293 -> [w302 w304]
              tunnel: [w302 w303] -> w290
              frame False {
                # "These are the remaining states (at the moment the error occured). States can be altered according to business logic."
                # "NOT SHUTTING DOWN"
              }
              frame True {
                # "Developer can decide to alter the states but should be aware that during the shutdown process, there are certain states that must be run for the SMO to properly shut itself (and this process) down. As such, one can add states to perform additional clean-ups, but should append the remaining state to be executed."
                # "SHUTTING DOWN"
                n102 = call <vilib>:"Add State(s) to Queue__jki_lib_state_machine.vi"("State(s) in (\"\")"=w304) -> ("States Out"=w303:string)  [unwired: 14 in]
              }
            }
            n103 = Bundle By Name(cluster=w291, "Core.Last Error.error"=w296) -> (w292:T8)
            n104 = call <vilib>:"Add State(s) to Queue__jki_lib_state_machine.vi"("State(s) in Front (\"\")"=w290, "State(s) in (\"\")"=w301) -> ("States Out"=w300:string)  [unwired: 13 in]
          }
          frame "Macro: Read UI Config" {
            # "Do not put any code in this frame.\n(It is a separator no-op. You can make a copy of this frame to create a new Macro frame)"
            n105 = call <vilib>:"Add State(s) to Queue__jki_lib_state_machine.vi"("State(s) in Front (\"\")"="Configuration: Initialize\nConfiguration: Read UI Config File\nUI: Update FP Controls" ("State(s) in Front (\"\")"), "State(s) in (\"\")"=w311) -> ("States Out"=w310:string)  [unwired: 13 in]
          }
          frame "Macro: Write UI Config" {
            # "Do not put any code in this frame.\n(It is a separator no-op. You can make a copy of this frame to create a new Macro frame)"
            n106 = call <vilib>:"Add State(s) to Queue__jki_lib_state_machine.vi"("State(s) in Front (\"\")"="Data: Set UI Cluster\nConfiguration: Write UI Config File" ("State(s) in Front (\"\")"), "State(s) in (\"\")"=w317) -> ("States Out"=w316:string)  [unwired: 13 in]
          }
          frame "Macro: Exit" {
            # "Exit Macro\n(This is called once, when the VI exits)"
            n107 = Unbundle By Name(w319) -> ("Core.Close Panel on Exit?"=w329:bool)
            n108 = Select(t="UI: Front Panel State >> Close", s=w329, f="" ("Empty String Constant")) -> (s? t:f=w326:string)
            n109 = call <vilib>:"Add State(s) to Queue__jki_lib_state_machine.vi"("State(s) in Front (\"\")"="Data: Cleanup\nEvents: Unregister\nProcess: Self Terminate", "State(s) in (\"\")"="Process: Sync", "State(s) at Back (\"\")"="Exit") -> ("States Out"=w321:string)  [unwired: 12 in]
            n110 = call <vilib>:"Add State(s) to Queue__jki_lib_state_machine.vi"("State(s) in Front (\"\")"="Action: Close\nMacro: Write UI Config", "State(s) in (\"\")"=w326, "State(s) at Back (\"\")"=w321) -> ("States Out"=w325:string)  [unwired: 12 in]
            n111 = call <vilib>:"Add State(s) to Queue__jki_lib_state_machine.vi"("State(s) in Front (\"\")"=w325, "State(s) in (\"\")"=w332) -> ("States Out"=w331:string)  [unwired: 13 in]
          }
          frame "---------- Process ----------" {
            # "Template Separator\n(You can make a copy of, or modify, this frame)"
            n112 = call <vilib>:"Add State(s) to Queue__jki_lib_state_machine.vi"("State(s) in (\"\")"=w337) -> ("States Out"=w336:string)  [unwired: 14 in]
          }
          frame "Process: Sync" {
            n113 = Unbundle By Name(w345) -> ("Instrument UI"=w341:refnum<class "Inst UI.Framework-Template.lvclass">)
            n114 = call <vilib>:"WaitOnProcessSync.vi"("error in (no error)"=w340, "SMO"=w341) -> ("error out"=w339:errorcluster, "Don't run?"=w344:bool)  [unwired: 7 in, 1 out]
            n115 = Select(t="Data: Cleanup\nEvents: Unregister\nExit", s=w344, f="" ("Empty String Constant")) -> (s? t:f=w338:string)
            n116 = call <vilib>:"Add State(s) to Queue__jki_lib_state_machine.vi"("State(s) in Front (\"\")"=w338, "State(s) in (\"\")"=w348) -> ("States Out"=w347:string)  [unwired: 13 in]
          }
          frame "Process: Self Terminate" {
            n117 = Unbundle By Name(w350) -> ("Instrument UI"=w349:refnum<class "Inst UI.Framework-Template.lvclass">)
            n118 = call <vilib>:"SelfTerminate.vi"("error in (no error)"=w352, "SMO in"=w349) -> ("error out"=w351:errorcluster)  [unwired: 8 in, 1 out]
            n119 = call <vilib>:"Add State(s) to Queue__jki_lib_state_machine.vi"("State(s) in (\"\")"=w355) -> ("States Out"=w354:string)  [unwired: 14 in]
          }
          frame "---------- Events ----------" {
            # "Template Separator\n(You can make a copy of, or modify, this frame)"
            n120 = call <vilib>:"Add State(s) to Queue__jki_lib_state_machine.vi"("State(s) in (\"\")"=w360) -> ("States Out"=w359:string)  [unwired: 14 in]
          }
          frame "Events: Register" {
            # "Expand to add\nmore events"
            # "Base Class Protected Events"
            n121 = Unbundle By Name(w374) -> ("Instrument UI"=w367:refnum<class "Inst UI.Framework-Template.lvclass">, "Instrument"=w366:refnum<class "Inst.Framework-Template.lvclass">)
            n122 = call <vilib>:"GetProtectedEvents.vi"("SMO"=w367) -> ("error out"=w370:errorcluster, "SMO Protected Events"=w372:T10)  [unwired: 8 in, 1 out]
            n123 = call <userlib>:"Instrument.GetPublicEvents.vi"("Instrument"=w366) -> ("error out"=w368:errorcluster, "Instrument Public Events"=w369:T11, "Instrument out"=w364:refnum<class "Inst.Framework-Template.lvclass">)  [unwired: 8 in]
            n124 = call "Inst.Framework-Template.GetPublicEvents.vi"("Inst.Framework-Template in"=w364) -> ("error out"=w363:errorcluster, "Inst.Framework-Template Public Events"=w365:T12)  [unwired: 8 in, 1 out]
            n125 = register-events(w372, w369, w365) -> (reference out=w373:refnum<event-registration>, error out=w362:errorcluster)  [unwired: 2 in]
            n126 = Merge Errors(w362, w363, w368, w370, w361) -> (w371:errorcluster)
            n127 = call <vilib>:"Add State(s) to Queue__jki_lib_state_machine.vi"("State(s) in (\"\")"=w376) -> ("States Out"=w375:string)  [unwired: 14 in]
          }
          frame "Events: Unregister" {
            n128 = Unregister For Events(event registration refnum=w379, error in=w378) -> (error out=w377:errorcluster)
            n129 = call <vilib>:"Add State(s) to Queue__jki_lib_state_machine.vi"("State(s) in (\"\")"=w382) -> ("States Out"=w381:string)  [unwired: 14 in]
          }
          frame "---------- Configuration ----------" {
            # "Do not put any code in this frame.\n(It is a separator no-op. You can make a copy of this frame to create a new UI frame)"
            n130 = call <vilib>:"Add State(s) to Queue__jki_lib_state_machine.vi"("State(s) in (\"\")"=w387) -> ("States Out"=w386:string)  [unwired: 14 in]
          }
          frame "Configuration: Initialize" {
            # "Do not put any code in this frame.\n(It is a separator no-op. You can make a copy of this frame to create a new UI frame)"
            n131 = Unbundle By Name(w395) -> ("Configuration"=w393:refnum<class "Configuration.lvclass">, "Instrument"=w394:refnum<class "Inst.Framework-Template.lvclass">)
            n132 = call <vilib>:"GetName.vi"("error in (no error)"=w397, "SMO"=w394) -> ("error out"=w396:errorcluster, "Name"=w398:string)  [unwired: 6 in, 2 out]
            n133 = call <userlib>:"Default Path.vi"("error in (no error)"=w396, "Folder Name [Application Name]"=w398, "Configuration in"=w393) -> ("error out"=w389:errorcluster, "Configuration out"=w392:refnum<class "Configuration.lvclass">)  [unwired: 7 in]
            n134 = call <userlib>:"Write Section.vi"("error in (no error)"=w389, "Section"="UI", "Configuration in"=w392) -> ("error out"=w388:errorcluster, "Configuration out"=w391:refnum<class "Configuration.lvclass">)  [unwired: 7 in]
            n135 = Bundle By Name(cluster=w395, "Configuration"=w391) -> (w399:T8)
            n136 = call <vilib>:"Add State(s) to Queue__jki_lib_state_machine.vi"("State(s) in (\"\")"=w402) -> ("States Out"=w401:string)  [unwired: 14 in]
          }
          frame "Configuration: Write UI Config File" {
            # "Do not put any code in this frame.\n(It is a separator no-op. You can make a copy of this frame to create a new Data frame)"
            n137 = Unbundle By Name(w407) -> ("Configuration"=w404:refnum<class "Configuration.lvclass">, "UI Cluster"=w406:T6)
            n138 = call <userlib>:"Write Configuration.vi"("error in (no error)"=w403, "Variant"=w406, "Configuration in"=w404) -> ("error out"=w405:errorcluster)  [unwired: 7 in, 1 out]
            n139 = call <vilib>:"Add State(s) to Queue__jki_lib_state_machine.vi"("State(s) in (\"\")"=w410) -> ("States Out"=w409:string)  [unwired: 14 in]
          }
          frame "Configuration: Read UI Config File" {
            # "Do not put any code in this frame.\n(It is a separator no-op. You can make a copy of this frame to create a new UI frame)"
            n140 = Unbundle By Name(w413) -> ("UI Cluster"=w416:T6, "Configuration"=w419:refnum<class "Configuration.lvclass">)
            n141 = call <userlib>:"Read Configuration.vi"("INI Fomatted Cluster Type"=w416, "error in (no error)"=w415, "Configuration in"=w419) -> ("error out"=w418:errorcluster, "Configuration"=w417:variant)  [unwired: 6 in, 1 out]
            n142 = Variant To Data(error in=w418, type=w416, Variant=w417) -> (data=w412:T6, error out=w414:errorcluster)
            n143 = Bundle By Name(cluster=w413, "UI Cluster"=w412) -> (w411:T8)
            n144 = call <vilib>:"Add State(s) to Queue__jki_lib_state_machine.vi"("State(s) in (\"\")"=w422) -> ("States Out"=w421:string)  [unwired: 14 in]
          }
          frame "---------- Action ----------" {
            n145 = Unbundle By Name(w424) -> ("Instrument"=w425:refnum<class "Inst.Framework-Template.lvclass">)
            n146 = Bundle By Name(cluster=w424, "Instrument"=w425) -> (w423:T8)
            n147 = call <vilib>:"Add State(s) to Queue__jki_lib_state_machine.vi"("State(s) in (\"\")"=w429) -> ("States Out"=w428:string)  [unwired: 14 in]
          }
          frame "Action: Notify UI Closed" {
            # "Notify that the UI has been closed"
            n148 = Unbundle By Name(w430) -> ("Instrument UI"=w433:refnum<class "Inst UI.Framework-Template.lvclass">)
            n149 = call <vilib>:"Hide.vi"("error in (no error)"=w432, "SMO.UI"=w433) -> ("error out"=w431:errorcluster)  [unwired: 8 in, 1 out]
            n150 = call <vilib>:"Add State(s) to Queue__jki_lib_state_machine.vi"("State(s) in (\"\")"=w436) -> ("States Out"=w435:string)  [unwired: 14 in]
          }
          frame "Action: getAll" {
            n151 = Unbundle By Name(w440) -> ("getAll"=w438:T5, "Instrument"=w443:refnum<class "Inst.Framework-Template.lvclass">)
            n152 = call "GET ALL.vim"("type"=w438, "error in (no error)"=w441, "Instrument in"=w443) -> ("error out"=w445:errorcluster, "getAll"=w437:T5, "Instrument out"=w439:refnum<class "Inst.Framework-Template.lvclass">)  [unwired: 6 in]
            n153 = Bundle By Name(cluster=w440, "Instrument"=w439, "getAll"=w437) -> (w442:T8)
            n154 = call <vilib>:"Add State(s) to Queue__jki_lib_state_machine.vi"("State(s) in Front (\"\")"="" ("State(s) in Front (\"\")"), "State(s) in (\"\")"=w448) -> ("States Out"=w447:string)  [unwired: 13 in]
          }
          frame "Action: Open" {
            n155 = Unbundle By Name(w455) -> ("Instrument"=w453:refnum<class "Inst.Framework-Template.lvclass">)
            n156 = call <userlib>:"Write Client Type.vi"("error in (no error)"=w450, "Client Type"=Client_Type--Enum."Local", "Instrument in"=w453) -> ("error out"=w451:errorcluster, "Instrument out"=w452:refnum<class "Inst.Framework-Template.lvclass">)  [unwired: 7 in]
            n157 = call-dynamic "Open.vi"("error in (no error)"=w451, "Inst.Framework-Template in"=w452) -> ("error out"=w458:errorcluster, "Inst.Framework-Template out"=w454:refnum<class "Inst.Framework-Template.lvclass">)  [unwired: 8 in]
            n158 = Bundle By Name(cluster=w455, "Instrument"=w454) -> (w456:T8)
            n159 = call <vilib>:"Add State(s) to Queue__jki_lib_state_machine.vi"("State(s) in Front (\"\")"="" ("State(s) in Front (\"\")"), "State(s) in (\"\")"=w461) -> ("States Out"=w460:string)  [unwired: 13 in]
          }
          frame "Action: Close" {
            n160 = Unbundle By Name(w463) -> ("Instrument"=w466:refnum<class "Inst.Framework-Template.lvclass">)
            n161 = call-dynamic "Close.vi"("error in (no error)"=w464, "Inst.Framework-Template in"=w466) -> ("error out"=w468:errorcluster, "Inst.Framework-Template out"=w462:refnum<class "Inst.Framework-Template.lvclass">)  [unwired: 8 in]
            n162 = Bundle By Name(cluster=w463, "Instrument"=w462) -> (w465:T8)
            n163 = call <vilib>:"Add State(s) to Queue__jki_lib_state_machine.vi"("State(s) in Front (\"\")"="" ("State(s) in Front (\"\")"), "State(s) in (\"\")"=w471) -> ("States Out"=w470:string)  [unwired: 13 in]
          }
          frame "Action: Send Message to Instrument" {
            # "Send a message (command, data, etc) to the Instrument:process.vi"
            n164 = Unbundle By Name(w476) -> ("Instrument"=w475:refnum<class "Inst.Framework-Template.lvclass">)  [unwired: 1 out]
            n165 = call <userlib>:"Instrument.MessageToProcess.vi"("error in (no error)"=w473, "Instrument"=w475) -> ("error out"=w472:errorcluster, "Instrument out"=w474:refnum<class "Inst.Framework-Template.lvclass">)  [unwired: 8 in]
            n166 = Bundle By Name(cluster=w476, "Instrument"=w474) -> (w477:T8)
            n167 = call <vilib>:"Add State(s) to Queue__jki_lib_state_machine.vi"("State(s) in Front (\"\")"="" ("State(s) in Front (\"\")"), "State(s) in (\"\")"=w481) -> ("States Out"=w480:string)  [unwired: 13 in]
          }
          frame "Action: Send Message to Child" {
            # "Send a message (command, data, etc) to the Instrument.Child:process.vi"
            n168 = Unbundle By Name(w486) -> ("Instrument"=w485:refnum<class "Inst.Framework-Template.lvclass">)  [unwired: 1 out]
            n169 = call "Inst.Framework-Template.MessageToProcess.vi"("error in (no error)"=w483, "Inst.Framework-Template in"=w485) -> ("error out"=w482:errorcluster, "Inst.Framework-Template out"=w484:refnum<class "Inst.Framework-Template.lvclass">)  [unwired: 8 in]
            n170 = Bundle By Name(cluster=w486, "Instrument"=w484) -> (w487:T8)
            n171 = call <vilib>:"Add State(s) to Queue__jki_lib_state_machine.vi"("State(s) in Front (\"\")"="" ("State(s) in Front (\"\")"), "State(s) in (\"\")"=w491) -> ("States Out"=w490:string)  [unwired: 13 in]
          }
        }
      }
    }
    frame Error {
    }
  }
  n172 = call-parent "Process.vi"("error in"=w5, "Instrument UI in"=w4) -> ("error out"=w2:errorcluster, "Instrument UI out"=→"Inst UI.Framework-Template out":refnum<class "Inst UI.Framework-Template.lvclass">)  [unwired: 8 in]
  n173 = Merge Errors(w2, w1) -> (→"error out":errorcluster)
